vi "serial.vi"() -> ()   [LabVIEW 2018]
panel:
  in  "state":enum16{"설정", "읽기", "쓰기", "종"}(ring)
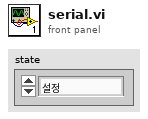
[diagram p1: front panel]
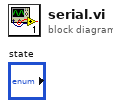
[diagram p0: block diagram]
diagram:
